vi "Spanfaktor in Tabelle schreiben.vi"   [LabVIEW 2015, in "Linearisierung v2.lvlib"]
uses:
  Linearisierung v2.lvlib
  Aktion Lin Daten aufarbeiten.ctl
  Seiten/FT-IR/Span/Spanfaktor.lvlib
  Seiten/FT-IR/Span/Aktion FGV Span.ctl
types:
  T1 = typedef "Linearisierung v2.lvlib/Aktion Lin Daten aufarbeiten.ctl" = enum16{"lesen", "Protkolldaten", "speichern", "laden", "EPA auswerten", "Tabelle schreiben", "Lin auswerten", "Tab init", "Stufentabelle", "EPA aktiviert", "Nachbehandlung laden", "Tabelle löschen", "Istwerte löschen", "Zeile löschen", "Zeile einfügen", "LIN aktiviert", "LIN/EPA aktiv laden", "EGAK Tab"}
  T2 = typedef "FT-IR.lvlib/Spanfaktor.lvlib/Aktion FGV Span.ctl" = enum16{"lesen", "schreiben", "Seite aktiv"}
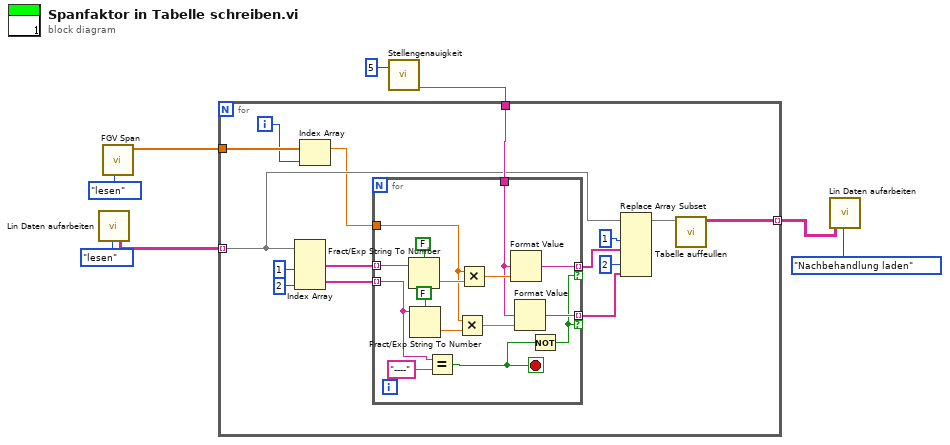
[diagram p0: block diagram]
diagram:
  n1 = call "Lin Daten aufarbeiten.vi"("Aktionen"=Aktion_Lin_Daten_aufarbeiten."lesen") -> ("TabellenArray"=w6:string[][][])  [unwired: 17 in, 9 out]
  n2 = call "FGV Span.vi"("Aktion"=Aktion_FGV_Span."lesen") -> ("Span"=w5:sgl[])  [unwired: 8 in, 2 out]
  n3 = call "Stellengenauigkeit.vi"("Genauigkeit (6)"=i16 5) -> ("Formatstring"=w3:string)  [unwired: 9 in, 1 out]
  n4 = for {
    tunnel: w6 -> [w17] mode=indexing
    tunnel: w5 -> [w19]
    tunnel: w3 -> [w18]
    tunnel: [w11] -> w1 mode=indexing
    i -> [w9]
    n5 = Index Array(array=w17, index (col) #1=1 ("Deaktivierter Index (Spalte)"), index (col) #2=2 ("Index (Spalte)")) -> (element #1=w22:string[], element #2=w20:string[])  [unwired: 2 in]
    n6 = Index Array(array=w19, index=w9) -> (element=w10:sgl)
    n7 = for {
      tunnel: w22 -> [w38] mode=indexing
      tunnel: w20 -> [w28] mode=indexing
      tunnel: w10 -> [w33]
      tunnel: w18 -> [w30]
      tunnel: [w27] -> w14 mode=indexing if=w25
      tunnel: [w26] -> w13 mode=indexing if=w25
      stop <- w24 stop-if-true
      n8 = Fract/Exp String To Number(use system decimal point (T)=FALSE ("Systemdezimalzeichen verwenden (T)"), string=w38) -> (number=w35:dbl)  [unwired: 2 in, 1 out]
      n9 = Fract/Exp String To Number(use system decimal point (T)=FALSE ("Systemdezimalzeichen verwenden (T)"), string=w28) -> (number=w34:dbl)  [unwired: 2 in, 1 out]
      n10 = Equal?(x=w28, y="----") -> (x = y?=w24:bool)
      n11 = Multiply(x=w33, y=w34) -> (x*y=w31:dbl)
      n12 = Multiply(x=w33, y=w35) -> (x*y=w32:dbl)
      n13 = Format Value(format string=w30, value (0)=w32) -> (output string=w27:string)  [unwired: 1 in]
      n14 = Format Value(format string=w30, value (0)=w31) -> (output string=w26:string)  [unwired: 1 in]
      n15 = Not(x=w24) -> (.not. x?=w25:bool)
    }
    n16 = Replace Array Subset(array=w17, new element #1=w14, index (col) #1=1 ("Deaktivierter Index (Spalte)"), new element #2=w13, index (col) #2=2 ("Index (Spalte)")) -> (w12:string[][])  [unwired: 2 in]
    n17 = call "Tabelle auffeullen.vi"("Neue Tabelle"=w12) -> ("Tabelle"=w11:string[][])  [unwired: 10 in]
  }
  n18 = call "Lin Daten aufarbeiten.vi"("TabellenArray"=w1, "Aktionen"=Aktion_Lin_Daten_aufarbeiten."Nachbehandlung laden") -> ()  [unwired: 16 in, 10 out]
